vi "14_Factorial.vi"() -> ()   [LabVIEW 2018]
panel:
  in  "Number Input":i32
  out "Factorial":dbl
  # "Develop a HMI to find factorial of a given number using while loop."
  # "===>"
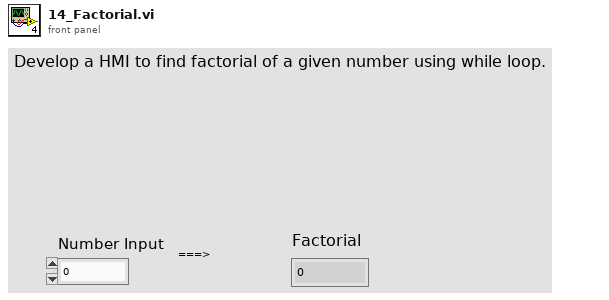
[diagram p1: front panel]
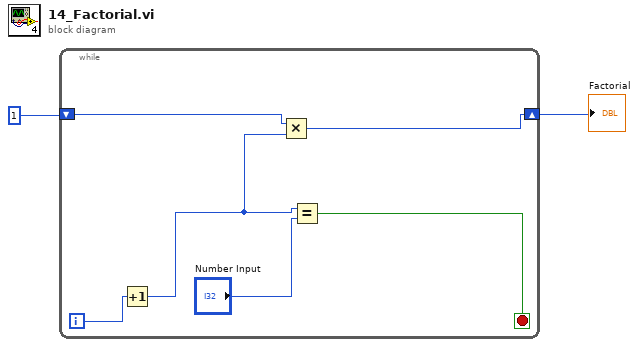
[diagram p0: block diagram]
diagram:
  n1 = while {
    shift-right: [w4] -> w1
    shift-left: 1 -> [w5]
    i -> [w8]
    stop <- w3 stop-if-true
    n2 = Increment(x=w8) -> (x+1=w6:i32)
    n3 = Multiply(x=w5, y=w6) -> (x*y=w4:i32)
    n4 = Equal?(x=w6, y="Number Input") -> (x = y?=w3:bool)
  }
  "Factorial" <- w1
